vi "TaskManager.vi"() -> ()   [LabVIEW 2016]
panel:
  out "Memory Usage":i32(graph)
  out "CPU Load":u8(slide) scale=0.0..100.0
  in  "Empty":bool
  in  "Process list":i32(listbox)
  in  "stop":bool
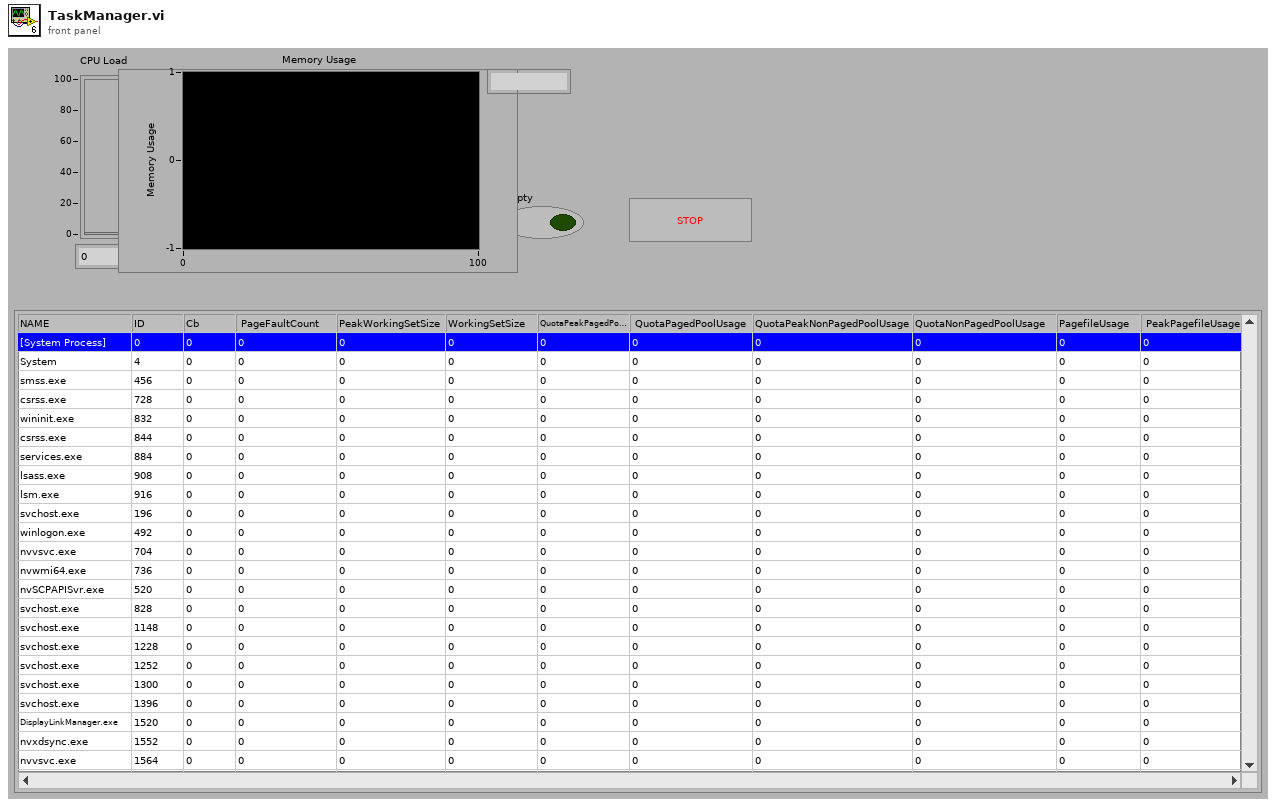
[diagram p1: front panel]
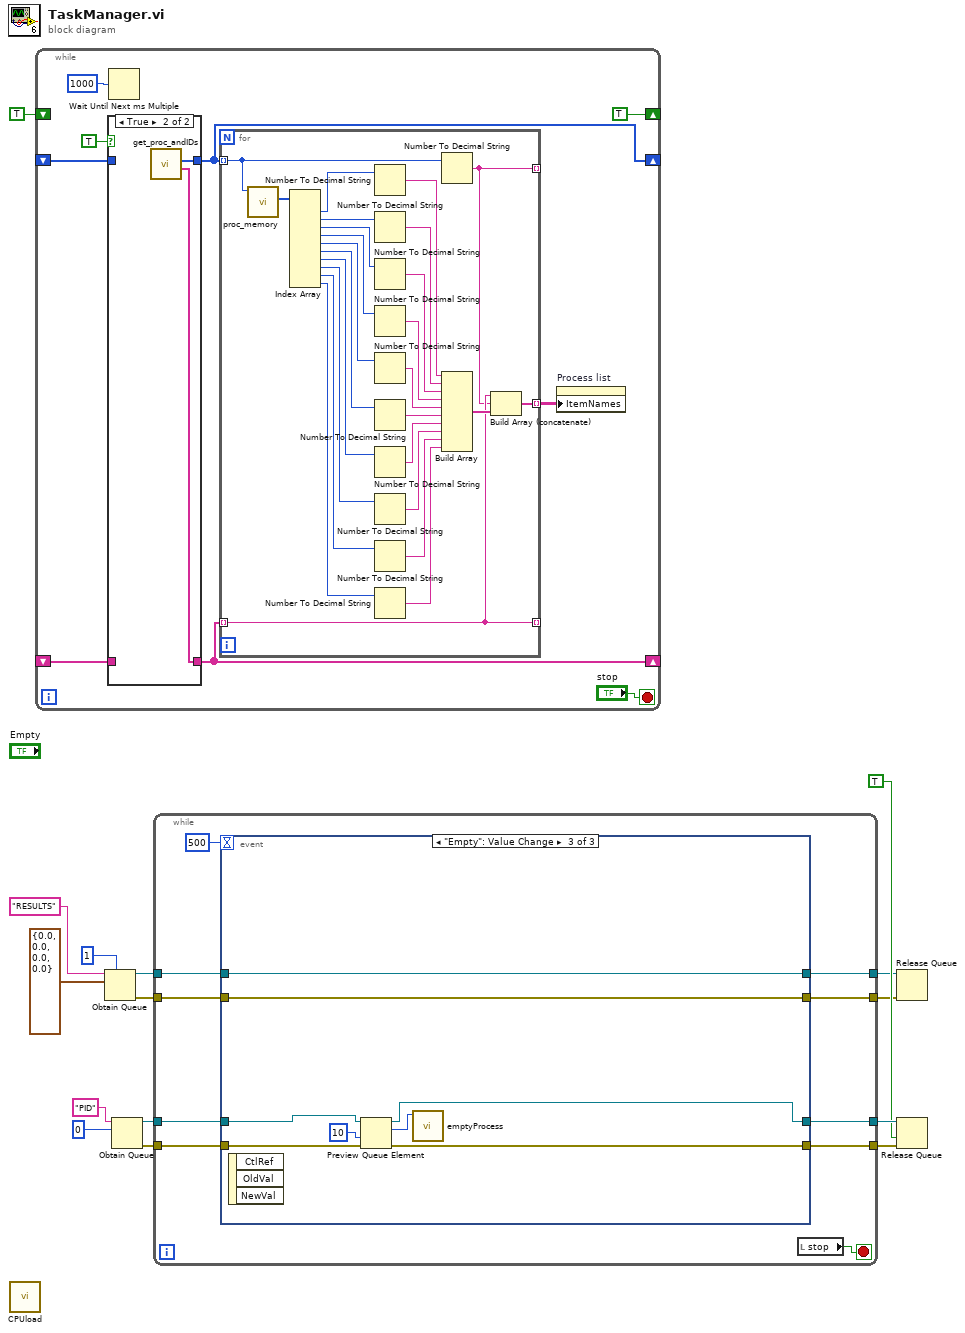
[diagram p0: block diagram]
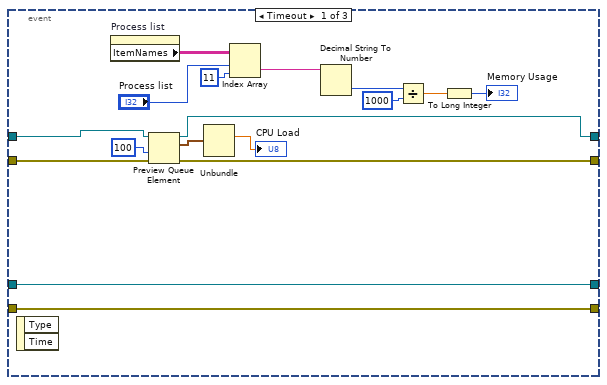
[diagram p2: hidden frame]
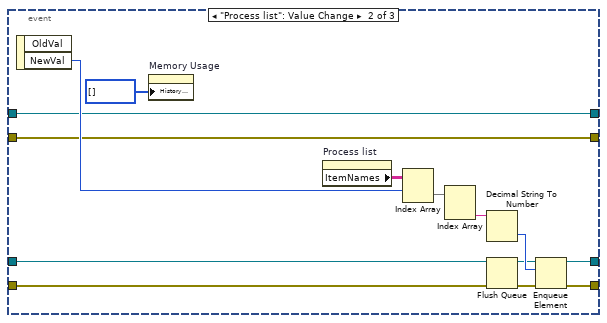
[diagram p3: hidden frame]
diagram:
  n1 = call "CPUload.vi"() -> ()  [unwired: 10 in, 2 out]
  n2 = while {
    shift-right: [w16] -> _
    shift-left: _ -> [w21]
    shift-right: [w20] -> _
    shift-left: _ -> [w19]
    shift-right: [TRUE] -> _
    shift-left: TRUE -> [_]
    stop <- "stop" stop-if-true
    n3 = case shown="True" TRUE {
      tunnel: [w26 w28] -> w16
      tunnel: [w25 w27] -> w20
      tunnel: w21 -> [w26 _]
      tunnel: w19 -> [w25 _]
      frame False {
      }
      frame True {
        n4 = call "get_proc_andIDs.vi"() -> ("procese"=w27:string[], "IDs 2"=w28:u32[])  [unwired: 10 out]
      }
    }
    n5 = Wait Until Next ms Multiple(millisecond multiple=u32 1000) -> ()  [unwired: 1 out]
    n6 = for {
      tunnel: w16 -> [w45] mode=indexing
      tunnel: w20 -> [w30] mode=indexing
      tunnel: [w44] -> w22 mode=indexing
      tunnel: [w30] -> _ mode=indexing
      tunnel: [w29] -> _ mode=indexing
      n7 = call "proc_memory.vi"("id"=w45) -> ("info 2"=w43:u32[])  [unwired: 10 out]
      n8 = Index Array(array=w43) -> (element #1=w42:u32, element #2=w41:u32, element #3=w40:u32, element #4=w39:u32, element #5=w38:u32, element #6=w37:u32, element #7=w36:u32, element #8=w35:u32, element #9=w34:u32, element #10=w33:u32)  [unwired: 10 in]
      n9 = Number To Decimal String(number=w42) -> (decimal integer string=w54:string)  [unwired: 1 out]
      n10 = Number To Decimal String(number=w41) -> (decimal integer string=w53:string)  [unwired: 1 out]
      n11 = Number To Decimal String(number=w40) -> (decimal integer string=w52:string)  [unwired: 1 out]
      n12 = Number To Decimal String(number=w39) -> (decimal integer string=w51:string)  [unwired: 1 out]
      n13 = Number To Decimal String(number=w38) -> (decimal integer string=w50:string)  [unwired: 1 out]
      n14 = Number To Decimal String(number=w37) -> (decimal integer string=w49:string)  [unwired: 1 out]
      n15 = Number To Decimal String(number=w36) -> (decimal integer string=w48:string)  [unwired: 1 out]
      n16 = Number To Decimal String(number=w35) -> (decimal integer string=w47:string)  [unwired: 1 out]
      n17 = Number To Decimal String(number=w34) -> (decimal integer string=w46:string)  [unwired: 1 out]
      n18 = Number To Decimal String(number=w33) -> (decimal integer string=w32:string)  [unwired: 1 out]
      n19 = Number To Decimal String(number=w45) -> (decimal integer string=w29:string)  [unwired: 1 out]
      n20 = Build Array(w54, w53, w52, w51, w50, w49, w48, w47, w46, w32) -> (w31:string[])
      n21 = Build Array (concatenate)(w30, w29, w31) -> (w44:string[])
    }
    n22 = property on="Process list" class="MCListbox (strict)"("ItemNames"=w22) -> ()  [unwired: 2 in, 2 out]
  }
  n23 = Obtain Queue(max queue size (-1, unlimited)=1, name (unnamed)="RESULTS", element data type=cluster{dbl, dbl, dbl, dbl} {0.0, 0.0, 0.0, 0.0}) -> (queue out=w7:refnum<queue>, error out=w6:errorcluster)  [unwired: 2 in, 1 out]
  n24 = Obtain Queue(name (unnamed)="PID", element data type=0) -> (queue out=w12:refnum<queue>, error out=w11:errorcluster)  [unwired: 3 in, 1 out]
  n25 = while {
    tunnel: w12 -> [w64]
    tunnel: w11 -> [w63]
    tunnel: w7 -> [w62]
    tunnel: w6 -> [w61]
    tunnel: [w58] -> w4
    tunnel: [w57] -> w5
    tunnel: [w56] -> w1
    tunnel: [w55] -> w2
    stop <- w60 stop-if-true
    n26 = event shown="[2] \"Empty\": Value Change" {
      selector: _ -> [_ _ _]
      dyn-events: _ -> [_ _ _]
      timeout: 500 -> [_ _ _]
      tunnel: w64 -> [w68 w86 w102]
      tunnel: w63 -> [w67 w85 w103]
      tunnel: w62 -> [w81 w88 w97]
      tunnel: w61 -> [w80 w87 w96]
      tunnel: [w68 w90 w99] -> w58
      tunnel: [w67 w89 w98] -> w57
      tunnel: [w66 w88 w97] -> w56
      tunnel: [w65 w87 w96] -> w55
      event Timeout {
        n27 = event-data() -> ()  [unwired: 1 in, 2 out]
        n28 = property on="Process list" class="MCListbox (strict)"() -> ("ItemNames"=w76:string[][])  [unwired: 2 in, 2 out]
        n29 = Preview Queue Element(queue=w81, timeout in ms (-1)=100, error in (no error)=w80) -> (queue out=w66:refnum<queue>, element=w78:cluster{dbl, dbl, dbl, dbl}, error out=w65:errorcluster)  [unwired: 1 out]
        n30 = Unbundle(w78) -> (→"CPU Load":dbl)  [unwired: 3 out]
        n31 = Index Array(array=w76, index (row)="Process list", index (col)=11 ("disabled index (col)")) -> (element=w73:string)
        n32 = Decimal String To Number(string=w73) -> (number=w72:i32)  [unwired: 2 in, 1 out]
        n33 = Divide(x=w72, y=1000) -> (x/y=w69:dbl)
        n34 = To Long Integer(number=w69) -> (32bit integer=→"Memory Usage":i32)
      }
      event "Process list": Value Change {
        n35 = event-data() -> ("NewVal"=w94:i32)  [unwired: 1 in, 1 out]
        n36 = property on="Memory Usage" class="WFChart (strict)"("History Data"=i32[] []) -> ()  [unwired: 2 in, 2 out]
        n37 = property on="Process list" class="MCListbox (strict)"() -> ("ItemNames"=w95:string[][])  [unwired: 2 in, 2 out]
        n38 = Index Array(array=w95, index (row)=w94) -> (element=w93:string[])  [unwired: 1 in]
        n39 = Index Array(array=w93) -> (element #2=w92:string)  [unwired: 2 in, 1 out]
        n40 = Decimal String To Number(string=w92) -> (number=w91:i32)  [unwired: 2 in, 1 out]
        n41 = Flush Queue(queue=w86, error in (no error)=w85) -> (queue out=w84:refnum<queue>, error out=w83:errorcluster)  [unwired: 1 out]
        n42 = Enqueue Element(queue=w84, element=w91, error in (no error)=w83) -> (queue out=w90:refnum<queue>, error out=w89:errorcluster)  [unwired: 1 in, 1 out]
      }
      event "Empty": Value Change {
        n43 = event-data() -> ()  [unwired: 1 in, 3 out]
        n44 = Preview Queue Element(queue=w102, timeout in ms (-1)=10, error in (no error)=w103) -> (queue out=w99:refnum<queue>, element=w100:i32, error out=w98:errorcluster)  [unwired: 1 out]
        n45 = call "emptyProcess.vi"("ID"=w100) -> ()  [unwired: 11 out]
      }
    }
    n46 = local read "stop"() -> (w60:bool)
  }
  n47 = Release Queue(queue=w1, error in (no error)=w2) -> ()  [unwired: 1 in, 3 out]
  n48 = Release Queue(queue=w4, force destroy? (F)=TRUE, error in (no error)=w5) -> ()  [unwired: 3 out]
